vi "CalVal-Analyze Data.vi"(0 "Data":dbl[][](array[numeric]), 1 "Navgs":i32, 5 "Params":T2, 7 "Test Freq (Hz)":dbl, 11 "error in (no error)":errorcluster) -> (6 "Update Data":T1, 15 "error out":errorcluster)   [LabVIEW 2020]
uses:
  Type Defs/CalVal-Params.ctl
  Utility VIs/Type Defs/Left-Right ring.ctl
  <vilib>/Analysis/baseanly.llb/Mean (DBL).vi
  Utility VIs/Math VIs/FFTtoR,Theta (1D).VI
  Utility VIs/Math VIs/Linear to dB (array).vi
  Utility VIs/Math VIs/Linear to dB (scalar).vi
  <vilib>/Analysis/NI_AALBase.lvlib
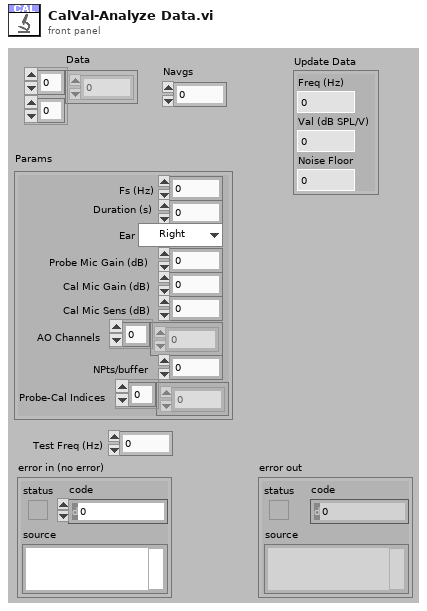
[diagram p1: front panel]
types:
  T1 = cluster{"Freq (Hz)":dbl, "Val (dB SPL/V)":dbl, "Noise Floor":dbl}
  T2 = typedef "CalVal-Params.ctl" = cluster{"Fs (Hz)":dbl, "Duration (s)":dbl, "Ear":T3, "Probe Mic Gain (dB)":dbl, "Cal Mic Gain (dB)":dbl, "Cal Mic Sens (dB)":dbl, "AO Channels":i32[], "NPts/buffer":i32, "Probe-Cal Indices":i32[]}
  T3 = typedef "Left-Right ring.ctl" = enum16{"Right", "Left"}
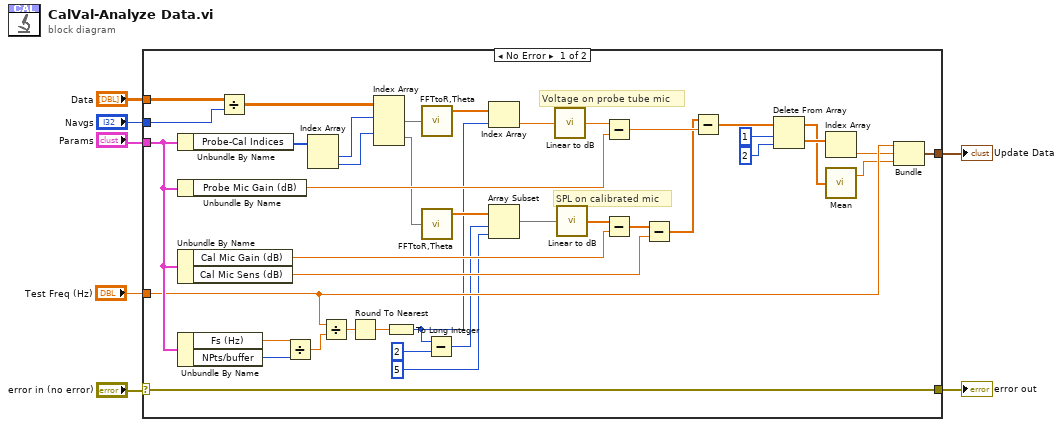
[diagram p0: block diagram]
diagram:
  n1 = case shown="No Error" "error in (no error)" {
    selector: "error in (no error)" -> [w47 w48]
    tunnel: [w47 w48] -> w6
    tunnel: "Data" -> [w46 _]
    tunnel: "Navgs" -> [w45 _]
    tunnel: "Params" -> [w29 _]
    tunnel: "Test Freq (Hz)" -> [w20 _]
    tunnel: [w19 _] -> w1
    frame No Error {
      # "SPL on calibrated mic"
      # "Voltage on probe tube mic"
      n2 = Unbundle By Name(w29) -> ("Probe-Cal Indices"=w44:i32[])
      n3 = Unbundle By Name(w29) -> ("Probe Mic Gain (dB)"=w36:dbl)
      n4 = Unbundle By Name(w29) -> ("Cal Mic Gain (dB)"=w40:dbl, "Cal Mic Sens (dB)"=w38:dbl)
      n5 = Unbundle By Name(w29) -> ("Fs (Hz)"=w28:dbl, "NPts/buffer"=w27:i32)
      n6 = Divide(x=w46, y=w45) -> (x/y=w33:dbl[][])
      n7 = Divide(x=w28, y=w27) -> (x/y=w26:dbl)
      n8 = Index Array(array=w44) -> (element #1=w43:i32, element #2=w42:i32)  [unwired: 2 in]
      n9 = Divide(x=w20, y=w26) -> (x/y=w31:dbl)
      n10 = Round To Nearest(number=w31) -> (nearest integer value=w30:dbl)
      n11 = Index Array(array=w33, index (row) #1=w43, index (row) #2=w42) -> (element #1=w23:dbl[], element #2=w32:dbl[])  [unwired: 2 in]
      n12 = To Long Integer(number=w30) -> (32bit integer=w8:i32)
      n13 = call-poly "FFTtoR,Theta.VI"("X"=w23) -> ("+Freq. Mag of FFT"=w21:dbl[])  [unwired: 1 in, 1 out]
      n14 = call-poly "FFTtoR,Theta.VI"("X"=w32) -> ("+Freq. Mag of FFT"=w22:dbl[])  [unwired: 1 in, 1 out]
      n15 = Subtract(x=w8, y=2) -> (x-y=w18:i32)
      n16 = Index Array(array=w21, index=w8) -> (element=w25:dbl)
      n17 = Array Subset(array=w22, index=w18, length=5) -> (w24:dbl[])
      n18 = call-poly "Linear to dB.vi"("Linear"=w25) -> ("dB"=w37:dbl)
      n19 = call-poly "Linear to dB.vi"("linear"=w24) -> ("dB"=w41:dbl[])
      n20 = Subtract(x=w37, y=w36) -> (x-y=w35:dbl)
      n21 = Subtract(x=w41, y=w40) -> (x-y=w39:dbl[])
      n22 = Subtract(x=w39, y=w38) -> (x-y=w34:dbl[])
      n23 = Subtract(x=w34, y=w35) -> (x-y=w15:dbl[])
      n24 = Delete From Array(array=w15, length=1, index=2) -> (deleted portion=w12:dbl[], array with subset deleted=w10:dbl[])
      n25 = Index Array(array=w12) -> (element=w11:dbl)  [unwired: 1 in]
      n26 = call-poly <vilib>:"Mean.vi"("X"=w10) -> ("mean"=w9:dbl)  [unwired: 1 out]
      n27 = Bundle("Test Freq (Hz)"=w20, w11, "mean"=w9) -> (w19:cluster{"Test Freq (Hz)":dbl, dbl, "mean":dbl})  [unwired: 1 in]
    }
    frame Error {
    }
  }
  "error out" <- w6
  "Update Data" <- w1
